vi "Get Z Factor.vi"(3 "X2":dbl, 4 "Xi":dbl, 5 "X1":dbl) -> (1 "Z":dbl)   [LabVIEW 2020]
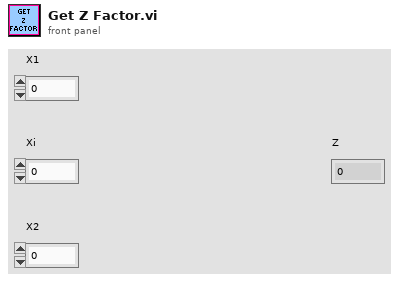
[diagram p1: front panel]
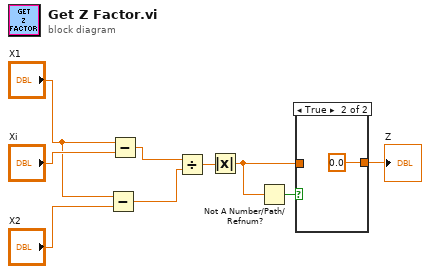
[diagram p0: block diagram]
diagram:
  n1 = Subtract(x="X1", y="X2") -> (x-y=w5:dbl)
  n2 = Subtract(x="X1", y="Xi") -> (x-y=w8:dbl)
  n3 = Divide(x=w8, y=w5) -> (x/y=w4:dbl)
  n4 = Absolute Value(x=w4) -> (abs(x)=w1:dbl)
  n5 = Not A Number/Path/Refnum?(number/path/refnum=w1) -> (NaN/Path/Refnum?=w3:bool)
  n6 = case shown="True" w3 {
    tunnel: w1 -> [w10 _]
    tunnel: [w10 0.0] -> w2
    frame False {
    }
    frame True {
    }
  }
  "Z" <- w2
